vi "期末-3.vi"() -> ()   [LabVIEW 2014]
uses:
  <vilib>/vision/NI_Vision_Development_Module.lvlib
panel:
  in  "Boolean":bool
  out "2":dbl[](array[numeric])
  out "最後":dbl[][](array[numeric])
  in  "填入飽和磁場分量尖點座標":dbl[](array[numeric])
  in  "最後分量值":dbl[](array[numeric])
  in  "Stop Button":bool
  out "0. 原始畫面":T1(plugin-control)
  in  "1. 範圍選擇":T2={"色相（H）"={0, 255}, "飽和度（S）"={0, 255}, "亮度（L）"={0, 255}} {"亮度（L）" scale=0.0..255.0; "飽和度（S）" scale=0.0..255.0; "色相（H）" scale=0.0..255.0}
  in  "3. Number of Erosion":i32=10
  out "Number of Particles":i32
  out "output cluster":cluster{"X":dbl, "Y":dbl}
  in  "顏色範圍初始化":bool
  in  "Tab Control":T3(tab)
  out "1. 顏色選取":T1(plugin-control)
  out "2. 填補空隙":T1(plugin-control)
  out "3. 移除雜點":T1(plugin-control)
  out "4. 形狀修正":T1(plugin-control)
  out "5. 選取結果":T1(plugin-control)
  out "Particle Measurements":dbl[][](array[numeric])
  out "Error Out":errorcluster
  in  "停止":bool
  out "瞬間尖點座標":dbl[][](array[numeric])
  out "滑鼠位置顏色":T4
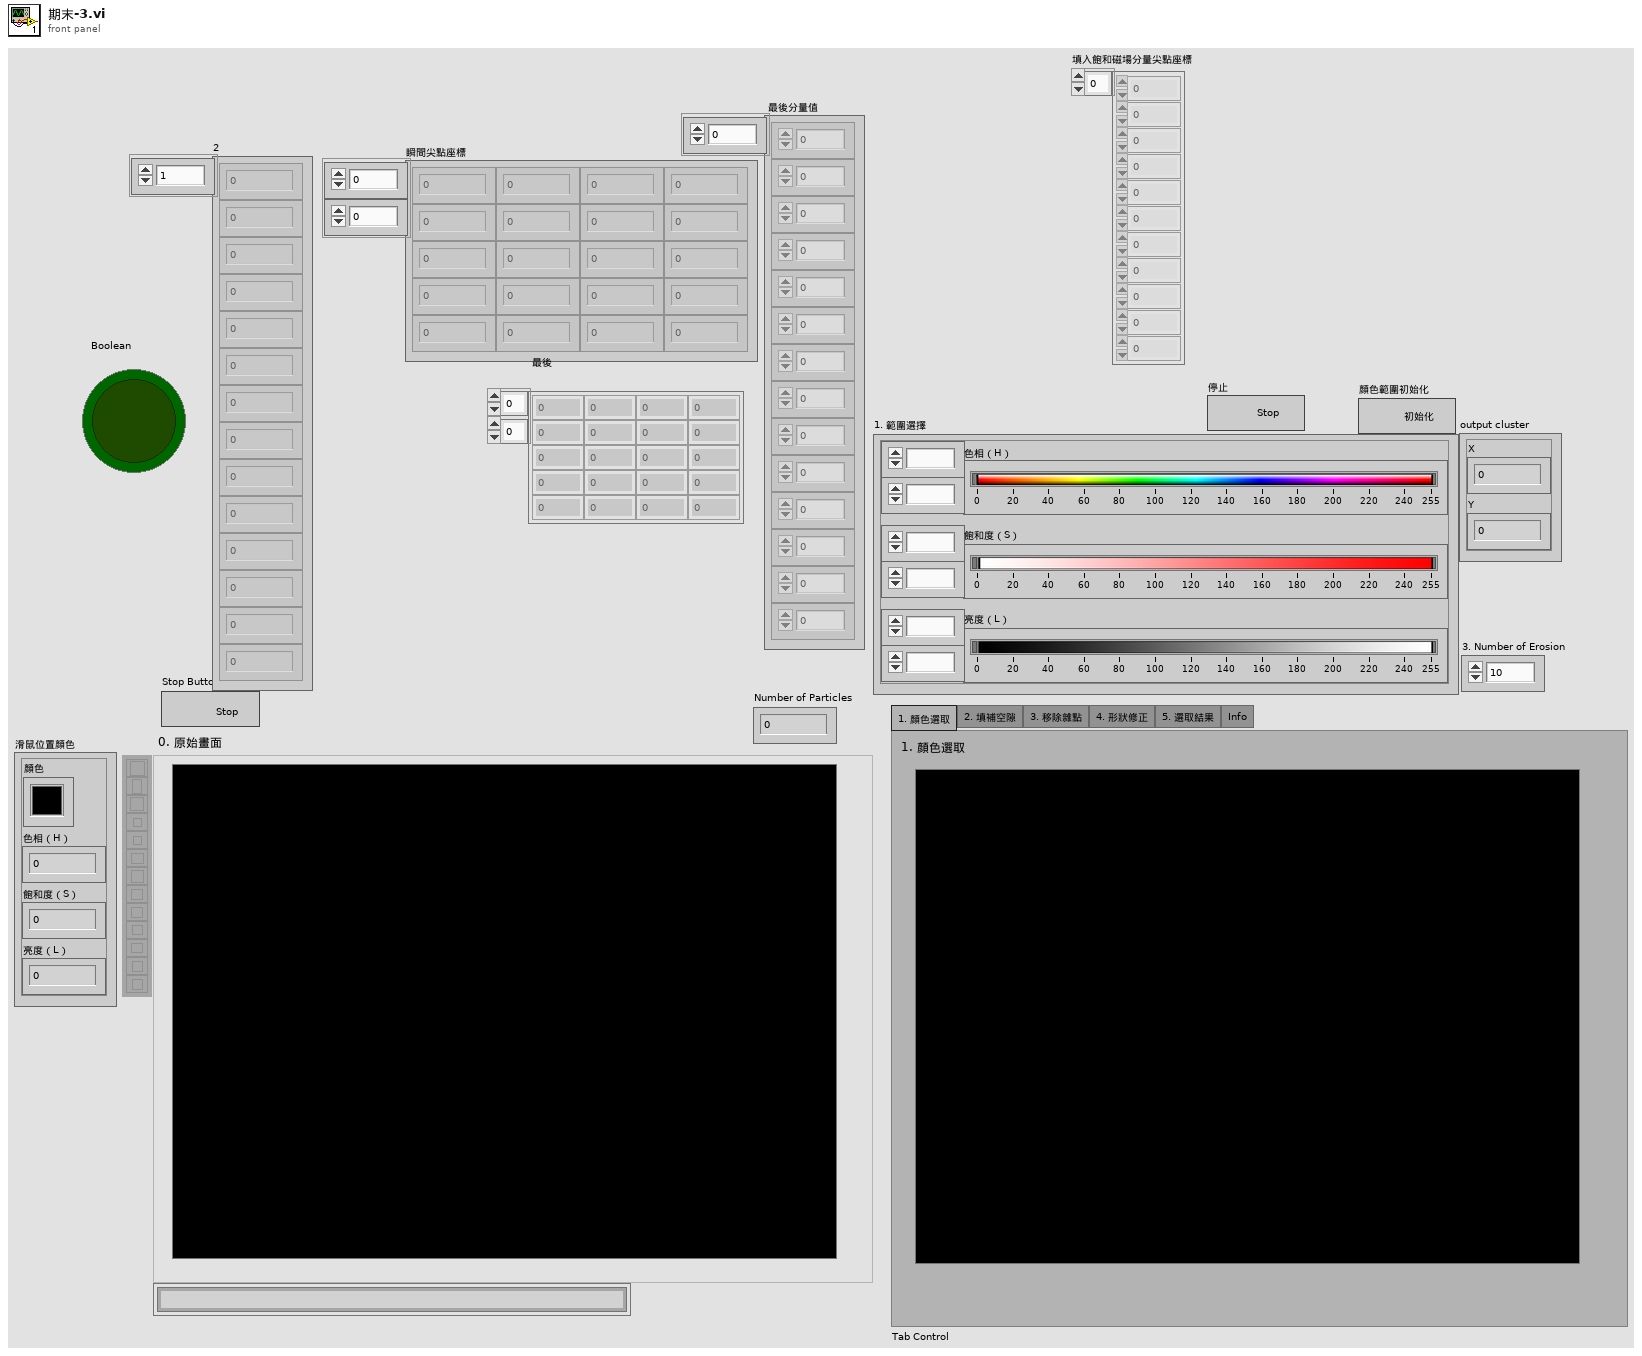
[diagram p1: front panel]
types:
  T1 = typedef "IMAQ Image.ctl" = refnum<image>
  T2 = cluster{"色相（H）":cluster{u8, u8}, "飽和度（S）":cluster{u8, u8}, "亮度（L）":cluster{u8, u8}}
  T3 = enum32{"1. 顏色選取", "2. 填補空隙", "3. 移除雜點", "4. 形狀修正", "5. 選取結果", "Info"}
  T4 = cluster{"色相（H）":u8, "飽和度（S）":u8, "亮度（L）":u8, "顏色":u32}
  T5 = cluster{"Numeric":dbl, "Numeric":dbl, "Numeric":dbl, "Numeric":dbl}
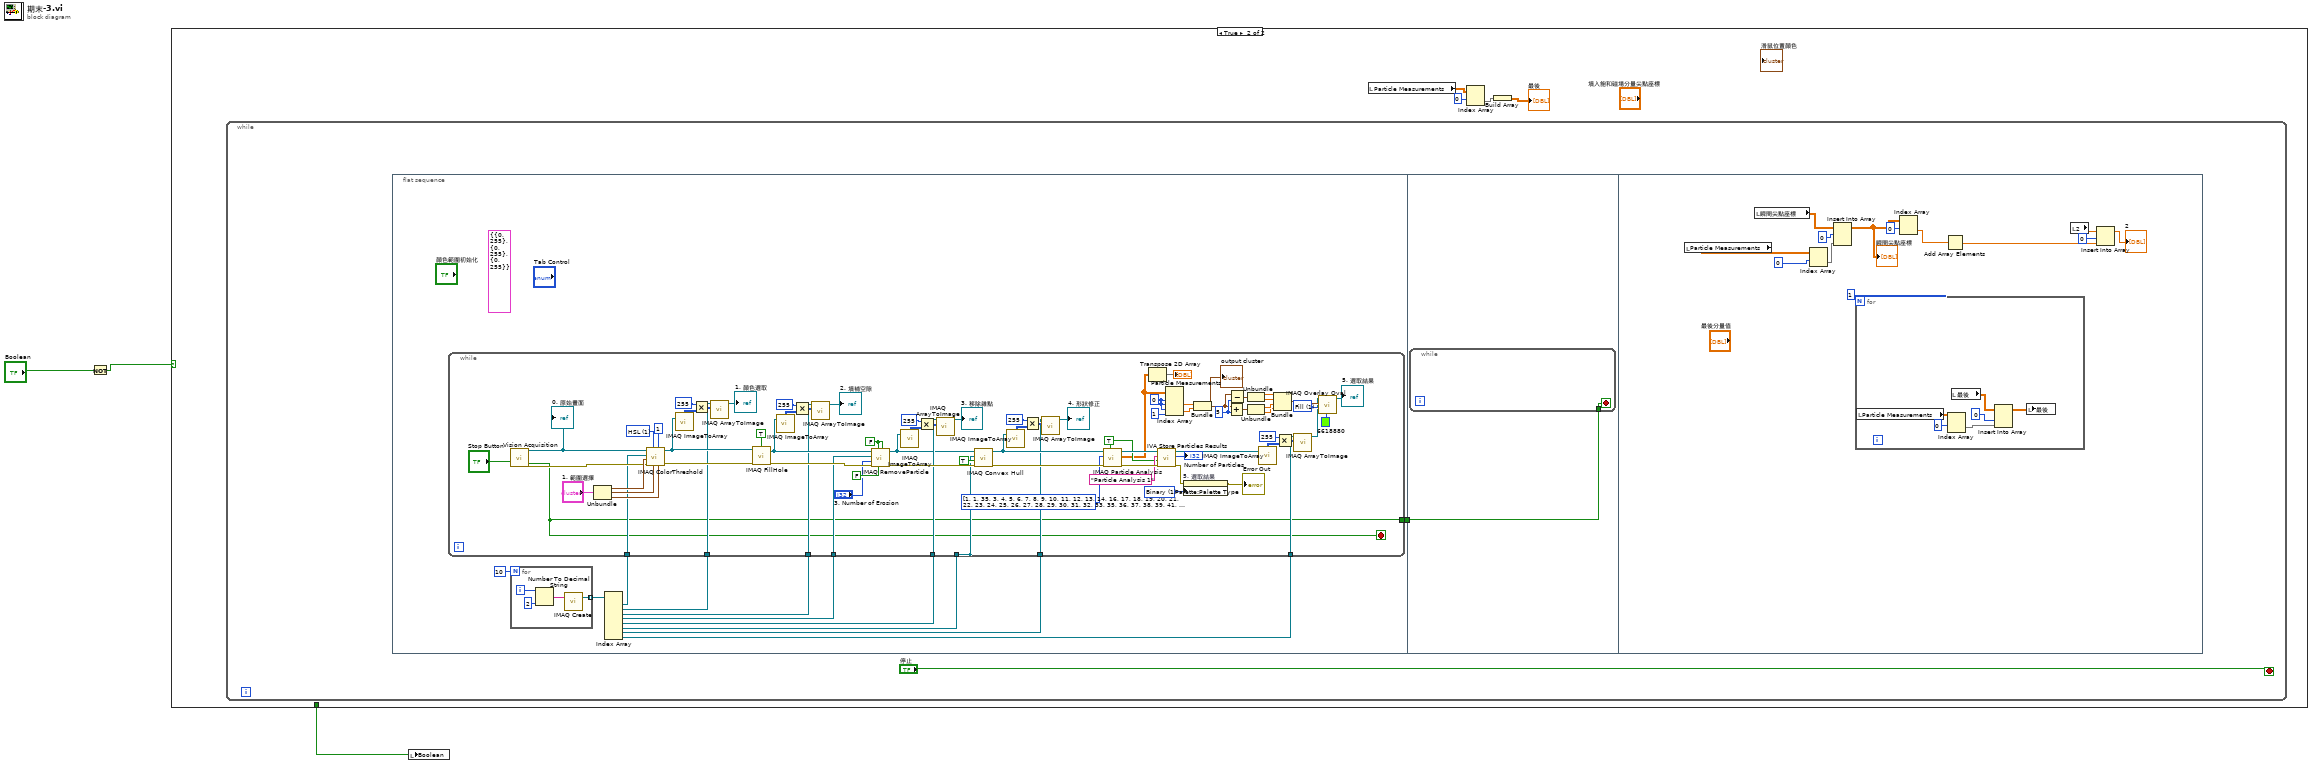
[diagram p0: block diagram]
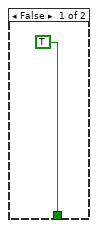
[diagram p2: hidden frame]
diagram:
  n1 = Not(x="Boolean") -> (.not. x?=w3:bool)
  n2 = case shown="True" w3 {
    tunnel: [TRUE _] -> w1
    frame False {
    }
    frame True {
      n3 = while {
        stop <- "停止" stop-if-true
        n4 = flat-sequence {
          tunnel: [w11] -> w10
          tunnel: w10 -> [w105]
          frame #0 {
            (unwired) T2 {"色相（H）"={0, 255}, "飽和度（S）"={0, 255}, "亮度（L）"={0, 255}} ("範圍選擇")
            n5 = for {
              N: 10 -> [_]
              tunnel: [w22] -> w21 mode=indexing
              i -> [w24]
              n6 = Number To Decimal String(number=w24, width (-)=2) -> (decimal integer string=w23:string)
              n7 = call "IMAQ Create"("Image Name"=w23) -> ("New Image"=w22:T1)  [unwired: 4 in, 1 out]
            }
            n8 = Index Array(array=w21) -> (element #1=w20:T1, element #2=w19:T1, element #3=w18:T1, element #4=w16:T1, element #5=w15:T1, element #6=w14:T1, element #7=w13:T1, element #8=w12:T1)  [unwired: 8 in]
            n9 = while {
              tunnel: w18 -> [w66]
              tunnel: w16 -> [w81]
              tunnel: w14 -> [w79]
              tunnel: [w79] -> _
              tunnel: w19 -> [w73]
              tunnel: w20 -> [w65]
              tunnel: w15 -> [w61]
              tunnel: w13 -> [w53]
              tunnel: w12 -> [w30]
              tunnel: [w26] -> w11
              stop <- w26 stop-if-true
              w35 = u32 1 items=["Frame", "Fill"] ("Drawing Mode (Frame)")
              w44 = 5
              w49 = 0
              w82 = u32 1 items=["Grayscale", "Binary", "Gradient", "Rainbow", "Temperature", "User Defined"] ("Palette")
              w91 = i32[] [1, 1, 35, 3, 4, 5, 6, 7, 8, 9, 10, 11, 12, 13, 14, 16, 17, 18, 19, 20, 21, 22, 23, 24, 25, 26, 27, 28, 29, 30, 31, 32, 33, 35, 36, 37, 38, 39, 41, 42, 43, 45, 46, 48, 49, 50, 51, 53, 54, 55, 56, 58, 59, 60, 61, 62, 63, 64, 65, 66, 68, 69, 70, 71, 72, 73, 74, 75, 76, 77, 78, 79, 80, 81, 82, 83, 84, 85, 86, 87, 88] items=["Center of Mass X", "Center of Mass Y", "First Pixel X", "First Pixel Y", "Bounding Rect Left", "Bounding Rect Top", "Bounding Rect Right", "Bounding Rect Bottom", "Max Feret Diameter Start X", "Max Feret Diameter Start Y", "Max Feret Diameter End X", "Max Feret Diameter End Y", "Max Horiz. Segment Length Left", "Max Horiz. Segment Length Right", "Max Horiz. Segment Length Row", "-", "Bounding Rect Width", "Bounding Rect Height", "Bounding Rect Diagonal", "Perimeter", "Convex Hull Perimeter", "Holes' Perimeter", "Max Feret Diameter", "Equivalent Ellipse Major Axis", "Equivalent Ellipse Minor Axis", "Equivalent Ellipse Minor Axis (Feret)", "Equivalent Rect Long Side", "Equivalent Rect Short Side", "Equivalent Rect Diagonal", "Equivalent Rect Short Side (Feret)", "Average Horiz. Segment Length", "Average Vert. Segment Length", "Hydraulic Radius", "Waddel Disk Diameter", "-", "Area", "Holes' Area", "Particle & Holes' Area", "Convex Hull Area", "Image Area", "-", "Number of Holes", "Number of Horiz. Segments", "Number of Vert. Segments", "-", "Orientation", "Max Feret Diameter Orientation", "-", "% Area/Image Area", "% Area/(Particle & Holes' Area)", "Ratio of Equivalent Ellipse Axes", "Ratio of Equivalent Rect Sides", "-", "Elongation Factor", "Compactness Factor", "Heywood Circularity Factor", "Type Factor", "-", "Sum X", "Sum Y", "Sum XX", "Sum XY", "Sum YY", "Sum XXX", "Sum XXY", "Sum XYY", "Sum YYY", "-", "Moment of Inertia XX", "Moment of Inertia XY", "Moment of Inertia YY", "Moment of Inertia XXX", "Moment of Inertia XXY", "Moment of Inertia XYY", "Moment of Inertia YYY", "Norm. Moment of Inertia XX", "Norm. Moment of Inertia XY", "Norm. Moment of Inertia YY", "Norm. Moment of Inertia XXX", "Norm. Moment of Inertia XXY", "Norm. Moment of Inertia XYY", "Norm. Moment of Inertia YYY", "Hu Moment 1", "Hu Moment 2", "Hu Moment 3", "Hu Moment 4", "Hu Moment 5", "Hu Moment 6", "Hu Moment 7"] ("Pixel Measurements")
              w93 = TRUE ("Connectivity 4/8 (8)")
              w72 = FALSE ("Connectivity 4/8 (8)")
              w102 = u16 1 items=["RGB", "HSL", "HSV", "HSI"] ("Color Mode")
              n10 = call "Vision Acquisition"("Stop (F)"="Stop Button") -> ("Image Out"=w104:T1, "Stopped"=w26:bool, "error out"=w97:errorcluster)  [unwired: 24 in]
              "0. 原始畫面" <- w104
              n11 = Unbundle("1. 範圍選擇") -> ("色相（H）"=w101:cluster{u8, u8}, "飽和度（S）"=w100:cluster{u8, u8}, "亮度（L）"=w99:cluster{u8, u8})
              n12 = call "IMAQ ColorThreshold"("Blue or Luma or Val or Inten Range"=w99, "Replace Value"=1, "Green or Sat Range"=w100, "Color Mode"=w102, "error in (no error)"=w97, "Red or Hue Range"=w101, "Image Dst"=w65, "Image Src"=w104) -> ("error out"=w84:errorcluster, "Image Dst Out"=w78:T1)  [unwired: 2 out]
              n13 = call "IMAQ ImageToArray"("Image"=w78) -> ("Image Pixels (U8)"=w76:u8[][])  [unwired: 3 in, 4 out]
              n14 = Multiply(x=255, y=w76) -> (x*y=w75:i32[][])
              n15 = call "IMAQ ArrayToImage"("Image Pixels (U8)"=w75, "Image"=w73) -> ("Image Out"=→"1. 顏色選取":T1)  [unwired: 8 in, 1 out]
              n16 = call "IMAQ FillHole"("error in (no error)"=w84, "Image Src"=w78, "Connectivity 4/8 (8)"=TRUE) -> ("error out"=w88:errorcluster, "Image Dst Out"=w67:T1)  [unwired: 1 in, 2 out]
              n17 = call "IMAQ ImageToArray"("Image"=w67) -> ("Image Pixels (U8)"=w70:u8[][])  [unwired: 3 in, 4 out]
              n18 = Multiply(x=255, y=w70) -> (x*y=w71:i32[][])
              n19 = call "IMAQ ArrayToImage"("Image Pixels (U8)"=w71, "Image"=w66) -> ("Image Out"=→"2. 填補空隙":T1)  [unwired: 8 in, 1 out]
              n20 = call "IMAQ RemoveParticle"("Connectivity 4/8 (8)"=w72, "Low Pass/High Pass (Low)"=FALSE, "Square/Hexa (Square)"=w72, "error in (no error)"=w88, "Number of Erosion"="3. Number of Erosion", "Image Dst"=w81, "Image Src"=w67) -> ("error out"=w89:errorcluster, "Image Dst Out"=w59:T1)  [unwired: 3 out]
              n21 = call "IMAQ ImageToArray"("Image"=w59) -> ("Image Pixels (U8)"=w63:u8[][])  [unwired: 3 in, 4 out]
              n22 = Multiply(x=255, y=w63) -> (x*y=w62:i32[][])
              n23 = call "IMAQ ArrayToImage"("Image Pixels (U8)"=w62, "Image"=w61) -> ("Image Out"=→"3. 移除雜點":T1)  [unwired: 8 in, 1 out]
              n24 = call "IMAQ Convex Hull"("error in (no error)"=w89, "Connectivity 4/8 (8)"=TRUE, "Image Dst"=w79, "Image Src"=w59) -> ("error out"=w92:errorcluster, "Image Dst Out"=w54:T1)  [unwired: 6 out]
              n25 = call "IMAQ ImageToArray"("Image"=w54) -> ("Image Pixels (U8)"=w57:u8[][])  [unwired: 3 in, 4 out]
              n26 = Multiply(x=255, y=w57) -> (x*y=w58:i32[][])
              n27 = call "IMAQ ArrayToImage"("Image Pixels (U8)"=w58, "Image"=w53) -> ("Image Out"=→"4. 形狀修正":T1)  [unwired: 8 in, 1 out]
              n28 = call "IMAQ Particle Analysis"("Connectivity 4/8 (8)"=w93, "error in (no error)"=w92, "Pixel Measurements"=w91, "Image"=w54) -> ("error out"=w96:errorcluster, "Particle Measurements (Pixels)"=w50:dbl[][], "Image Out (duplicate)"=w94:T1)  [unwired: 1 in, 4 out]
              n29 = Transpose 2D Array(2D array=w50) -> (transposed array=→"Particle Measurements":dbl[][])
              n30 = call <vilib>:"IVA Store Particles Results.vi"("error in (no error)"=w96, "Connectivity 4/8 (8)"=w93, "Step Name"="Particle Analysis 1", "Image in"=w94) -> ("error out"=w83:errorcluster, "Number of Particles"=→"Number of Particles":i32, "Image dup"=w34:T1)  [unwired: 5 out]
              n31 = Index Array(array=w50, index (row) #1=w49, index (col) #1=w49, index (row) #2=w49, index (col) #2=1) -> (element #1=w47:dbl, element #2=w46:dbl)
              n32 = property on="5. 選取結果" class="ImageControl"(error in=w83, "Palette:Palette Type"=w82) -> (error out=→"Error Out":errorcluster)  [unwired: 1 in, 1 out]
              n33 = Bundle("Numeric"=w47, "Numeric"=w46) -> (w43:cluster{"Numeric":dbl, "Numeric":dbl})  [unwired: 1 in]
              "output cluster" <- w43
              n34 = Add(x=w43, y=w44) -> (x+y=w41:cluster{"Numeric":dbl, "Numeric":dbl})
              n35 = Subtract(x=w43, y=w44) -> (x-y=w42:cluster{"Numeric":dbl, "Numeric":dbl})
              n36 = Unbundle(w42) -> ("Numeric"=w40:dbl, "Numeric"=w39:dbl)
              n37 = Unbundle(w41) -> ("Numeric"=w38:dbl, "Numeric"=w37:dbl)
              n38 = call "IMAQ ImageToArray"("Image"=w34) -> ("Image Pixels (U8)"=w31:u8[][])  [unwired: 3 in, 4 out]
              n39 = Bundle("Numeric"=w40, "Numeric"=w39, "Numeric"=w38, "Numeric"=w37) -> (w36:T5)  [unwired: 1 in]
              n40 = Multiply(x=255, y=w31) -> (x*y=w32:i32[][])
              n41 = call "IMAQ ArrayToImage"("Image Pixels (U8)"=w32, "Image"=w30) -> ("Image Out"=w29:T1)  [unwired: 8 in, 1 out]
              n42 = call "IMAQ Overlay Oval"("Color"=u32 6618880, "Drawing Mode (Frame)"=w35, "Bounding Rectangle"=w36, "Image"=w29) -> ("Image Out"=→"5. 選取結果":T1)  [unwired: 6 in, 1 out]
            }
          }
          frame #1 {
            n43 = while {
              tunnel: w105 -> [w106]
              stop <- w106 stop-if-true
            }
          }
          frame #2 {
            n44 = local read "Particle Measurements"() -> (w117:dbl[][])
            n45 = local read "瞬間尖點座標"() -> (w111:dbl[][])
            n46 = Index Array(array=w117, index (row)=0) -> (element=w112:dbl[])  [unwired: 1 in]
            n47 = Insert Into Array "Insert Into Array"(array=w111, index (row)=0 ("index"), new element=w112) -> (w109:dbl[][])  [unwired: 1 in]
            "瞬間尖點座標" <- w109
            n48 = for {
              N: 1 -> [_]
              n49 = local read "Particle Measurements"() -> (w123:dbl[][])
              n50 = Index Array "Index Array"(array=w123, index (row)=0) -> (element=w121:dbl[])  [unwired: 1 in]
              n51 = local read "最後"() -> (w125:dbl[][])
              n52 = Insert Into Array "Insert Into Array"(array=w125, index (col)=0 ("index"), new element=w121) -> (w124:dbl[][])  [unwired: 1 in]
              n53 = local write "最後"(w124) -> ()
            }
            n54 = Index Array(array=w109, index (row)=0) -> (element=w107:dbl[])  [unwired: 1 in]
            n55 = Add Array Elements(numeric array=w107) -> (sum=w114:dbl)
            n56 = local read "2"() -> (w116:dbl[])
            n57 = Insert Into Array "Insert Into Array"(array=w116, index=0 ("index (row)"), new element=w114) -> (→"2":dbl[])
          }
        }
      }
      n58 = local read "Particle Measurements"() -> (w6:dbl[][])
      n59 = Index Array(array=w6, index (row)=0 ("index")) -> (element=w7:dbl[])  [unwired: 1 in]
      n60 = Build Array(w7) -> (→"最後":dbl[][])
    }
  }
  n61 = local write "Boolean"(w1) -> ()
